vi "ABB Extract Results.vi"(8 "Column#":i32[](array[numeric]), 9 "test results":dbl[][](array[numeric]), 10 "ID group":string[](array[string]), 11 "Report in":string) -> (1 "Report Out":string)   [LabVIEW 2017]
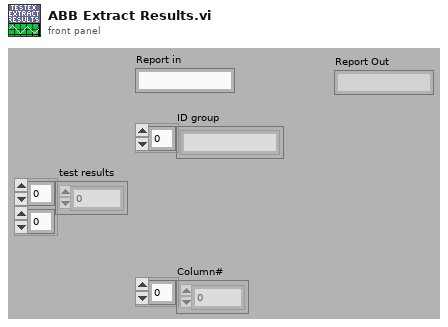
[diagram p1: front panel]
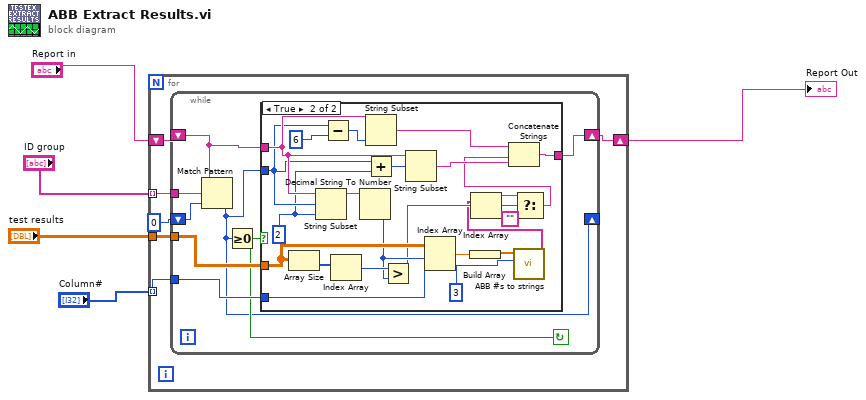
[diagram p0: block diagram]
diagram:
  n1 = for {
    tunnel: "test results" -> [w10]
    tunnel: "ID group" -> [w11] mode=indexing
    tunnel: "Column#" -> [w9] mode=indexing
    shift-right: [w7] -> w5
    shift-left: "Report in" -> [w8]
    n2 = while {
      tunnel: w11 -> [w19]
      tunnel: w10 -> [w18]
      tunnel: w9 -> [w17]
      shift-right: [w16] -> w7
      shift-left: w8 -> [w12]
      shift-right: [w13] -> _
      shift-left: 0 ("offset past match") -> [w14]
      stop <- w15 continue-if-true
      n3 = Match Pattern(string=w12, regular expression=w19, offset (0)=w14) -> (offset past match=w13:i32)  [unwired: 3 out]
      n4 = Greater Or Equal To 0?(x=w13) -> (x >= 0?=w15:bool)
      n5 = case shown="True" w15 {
        tunnel: w18 -> [_ w32]
        tunnel: w17 -> [_ w33]
        tunnel: w12 -> [w20 w36]
        tunnel: w13 -> [_ w35]
        tunnel: [w20 w40] -> w16
        frame False {
        }
        frame True {
          w34 = 2 ("length (rest)")
          n6 = Array Size(array=w32) -> (size(s)=w31:i32[])
          n7 = String Subset(string=w36, offset (0)=w35, length (rest)=w34) -> (substring=w43:string)
          n8 = Subtract(x=w35, y=6) -> (x-y=w38:i32)
          n9 = Index Array(array=w31) -> (element=w30:i32)  [unwired: 1 in]
          n10 = Decimal String To Number(string=w43) -> (number=w29:i32)  [unwired: 2 in, 1 out]
          n11 = String Subset(string=w36, length (rest)=w38) -> (substring=w37:string)  [unwired: 1 in]
          n12 = Add(x=w35, y=w34) -> (x+y=w42:i32)
          n13 = Greater?(x=w30, y=w29) -> (0:w28:bool)
          n14 = String Subset(string=w36, offset (0)=w42) -> (substring=w41:string)  [unwired: 1 in]
          n15 = Index Array(array=w32, index (row)=w29, index (col)=w33) -> (element=w24:dbl)
          n16 = Build Array(w24) -> (w23:dbl[])
          n17 = call "ABB #s to strings.vi"("Precision"=i16 3 ("precision (6)"), "Numbers in"=w23) -> ("Strings out"=w22:string[])  [unwired: 9 in]
          n18 = Index Array(array=w22) -> (element=w21:string)  [unwired: 1 in]
          n19 = Select(t=w21, s=w28, f="") -> (s? t:f=w27:string)
          n20 = Concatenate Strings(w37, w27, w41) -> (w40:string)
        }
      }
    }
  }
  "Report Out" <- w5
